vi "xxxxx.vi"(11 "xxxxx in":refnum<class "xxxxx.lvclass">) -> (3 "xxxxx out":refnum<class "xxxxx.lvclass">)   [LabVIEW 2021, in "Providers.lvlib" / "jettl Msg xxxxx.lvlib" / "xxxxx.lvclass"]
uses:
  xxxxx.lvclass
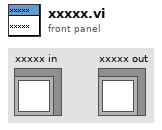
[diagram p1: front panel]
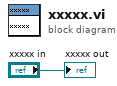
[diagram p0: block diagram]
diagram:
  "xxxxx out" <- "xxxxx in"
